vi "DevSysInfo (Read).vi"(6 "ISOBUS address":T1=-1 caption="ISOBUS address (-1)", 8 "error in":errorcluster, 10 "Device Identifier":string, 11 "Mercury Reference In":T2) -> (0 "error out":errorcluster, 2 "Device Sys Info":string[](array[string]), 3 "Mercury Reference Out":T2)   [LabVIEW 2013, in "Mercury iXX.lvlib" / "Pressure.lvlib"]
doc: "Returns the hardware version of the selected pressure device."
uses:
  <instrlib>/Mercury iXX/Public/Libraries/Pressure.lvlib
  <instrlib>/Mercury iXX/Public/Controls/Mercury Reference.ctl
  <instrlib>/Mercury iXX/Public/Controls/Comms Transport Layer.ctl
  <instrlib>/Mercury iXX/Private/Controls/Query Dynamic Reference.ctl
  <instrlib>/Mercury iXX/Public/Controls/ISOBus Address.ctl
  <instrlib>/Mercury iXX/Public/Libraries/System/Open/Open Device.vi
  <instrlib>/Mercury iXX/Public/Libraries/Pressure/Configuration/Read/HVer (Read).vi
  <instrlib>/Mercury iXX/Public/Libraries/Pressure/Configuration/Read/FVer (Read).vi
  <instrlib>/Mercury iXX/Public/Libraries/Pressure/Configuration/Read/Serial Number (Read).vi
  <instrlib>/Mercury iXX/Public/Libraries/Pressure/Configuration/Read/Nickname (Read).vi
  <instrlib>/Mercury iXX/Mercury iXX.lvlib
  <instrlib>/Mercury iXX/Public/Libraries/System.lvlib
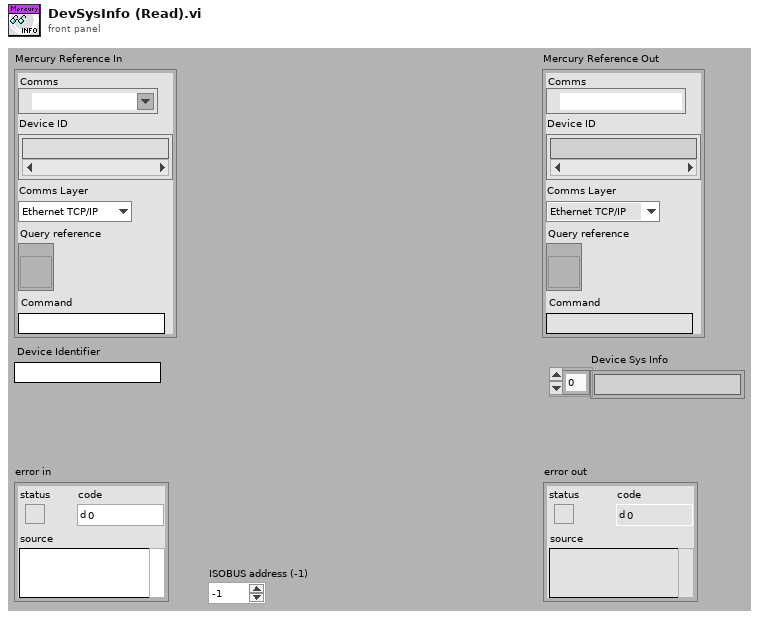
[diagram p1: front panel]
types:
  T1 = typedef "Mercury iXX.lvlib/ISOBus Address.ctl" = i32
  T2 = typedef "Mercury iXX.lvlib/Mercury Reference.ctl" = cluster{"Comms":refnum<visa-resource-name>, "Device ID":string[], "Comms Layer":T3, "Command":string, "Query reference":T4}
  T3 = typedef "Mercury iXX.lvlib/Comms Transport Layer.ctl" = enum16{"Ethernet TCP/IP", "USB", "ISOBus - RS-232", "GPIB"}
  T4 = typedef "Mercury iXX.lvlib/Query Dynamic Reference.ctl" = refnum<vi>
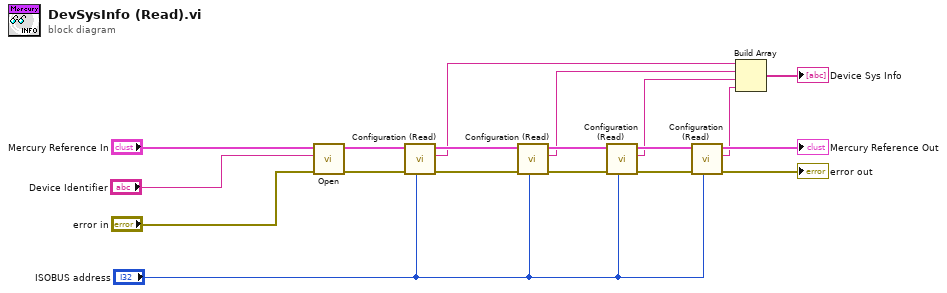
[diagram p0: block diagram]
diagram:
  n1 = call-poly <instrlib>:"Open.vi"("error in (no error)"="error in", "Device Identifier"="Device Identifier", "Mercury Reference In"="Mercury Reference In") -> ("error out"=w15:errorcluster, "Mercury Reference Out"=w16:T2)  [unwired: 1 in, 6 out]
  n2 = call-poly <instrlib>:"Configuration (Read).vi"("ISOBUS address"="ISOBUS address", "error in"=w15, "Mercury Reference In"=w16) -> ("error out"=w13:errorcluster, "Hardware Version"=w5:string, "Mercury Reference Out"=w14:T2)  [unwired: 6 out]
  n3 = call-poly <instrlib>:"Configuration (Read).vi"("ISOBUS address"="ISOBUS address", "error in"=w13, "Mercury Reference In"=w14) -> ("error out"=w11:errorcluster, "Firmware Version"=w4:string, "Mercury Reference Out"=w12:T2)  [unwired: 6 out]
  n4 = call-poly <instrlib>:"Configuration (Read).vi"("ISOBUS address"="ISOBUS address", "error in"=w11, "Mercury Reference In"=w12) -> ("error out"=w9:errorcluster, "Serial Number"=w3:string, "Mercury Reference Out"=w10:T2)  [unwired: 6 out]
  n5 = call-poly <instrlib>:"Configuration (Read).vi"("ISOBUS address"="ISOBUS address", "error in"=w9, "Mercury Reference In"=w10) -> ("error out"=→"error out":errorcluster, "Nickname"=w2:string, "Mercury Reference Out"=→"Mercury Reference Out":T2)  [unwired: 6 out]
  n6 = Build Array(w5, w4, w3, w2) -> (→"Device Sys Info":string[])
